vi "_Main.vi"   [LabVIEW 2017, in "Arm.lvlib"]
uses:
  Arm.lvlib
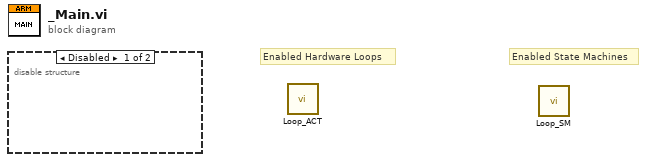
[diagram p0: block diagram]
diagram:
  # "Enabled State Machines"
  # "Enabled Hardware Loops"
  n1 = disable-structure shown="Disabled" {
    frame Disabled {
    }
    frame Enabled {
    }
  }
  n2 = call "Loop_ACT.vi"() -> ()  [unwired: 12 in]
  n3 = call "Loop_SM.vi"() -> ()  [unwired: 12 in]
